vi "Correct_Paths_For_OS_in_XML.vi"(2 "XML Elements":string) -> (0 "String":string)   [LabVIEW 2011]
uses:
  <vilib>/regexp/Match Regular Expression.xnode
panel:
  out "before match":string
  out "Numeric":i32
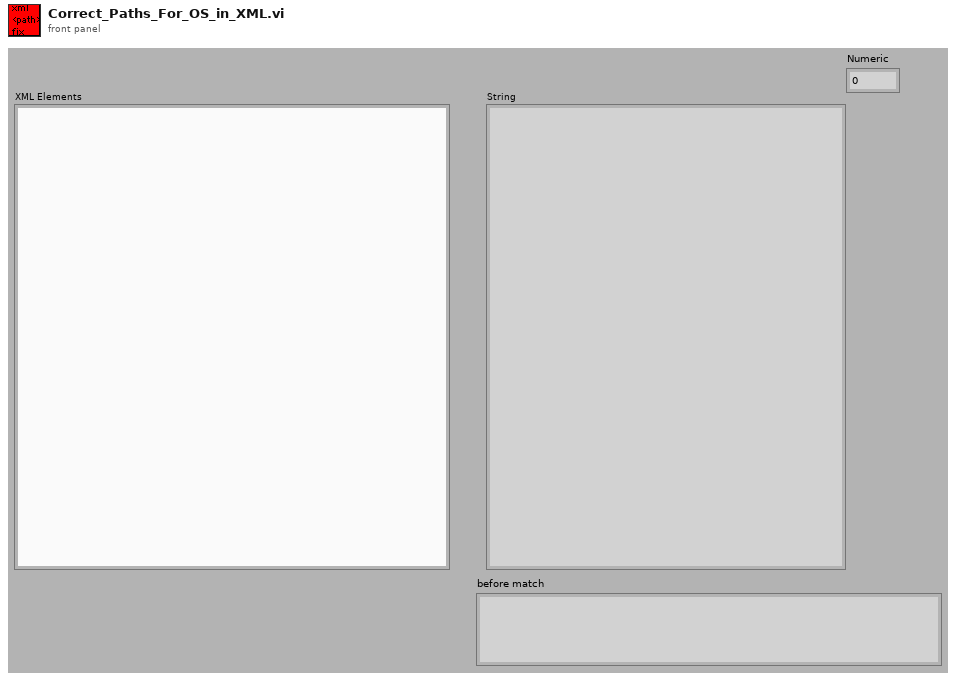
[diagram p1: front panel]
types:
  T1 = enum32{"invalid OS target", "Mac OS", "Windows 3.1", "Windows 95/NT", "Solaris 1", "Solaris 2", "HP-UX", "PowerMAX", "Linux", "Irix", "Rhapsody", "BeOS", "AIX", "OSF1", "VxWorks", "PharLap", "Carbon", "RTX", "Windows x64", "Linux x64"}
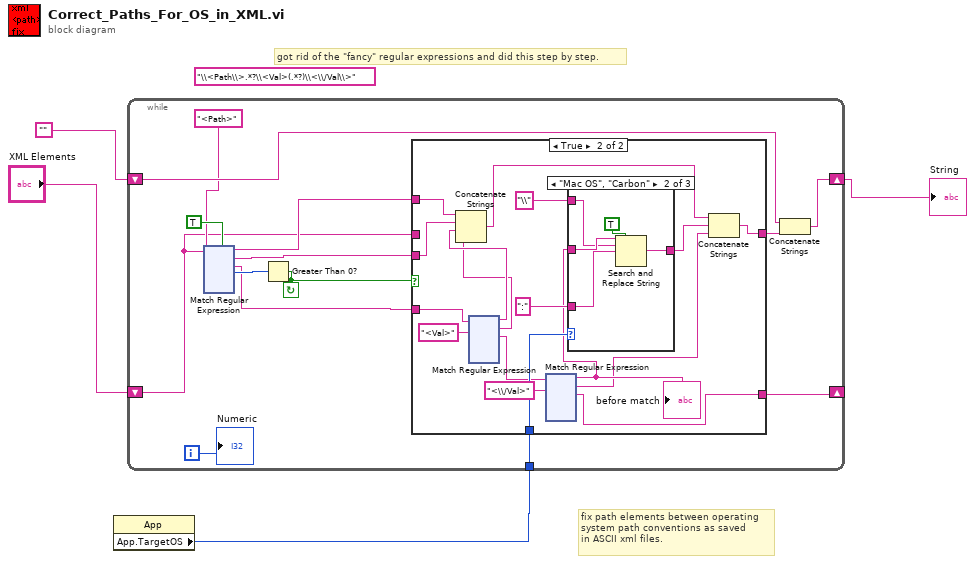
[diagram p0: block diagram]
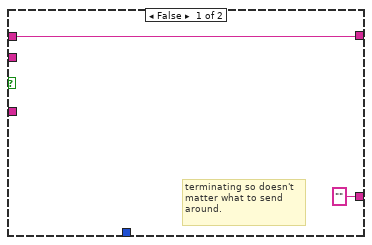
[diagram p2: hidden frame]
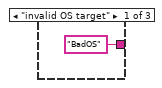
[diagram p3: hidden frame]
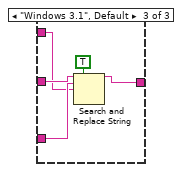
[diagram p4: hidden frame]
diagram:
  (unwired) "\\<Path\\>.*?\\<Val>(.*?)\\<\\/Val\\>"
  # "got rid of the \"fancy\" regular expressions and did this step by step."
  # "fix path elements between operating\nsystem path conventions as saved\nin ASCII xml files."
  n1 = property class="App"() -> ("App.TargetOS"=w2:T1)  [unwired: 2 in, 2 out]
  n2 = while {
    tunnel: w2 -> [w16]
    shift-right: [w5] -> _
    shift-left: "XML Elements" -> [w7]
    shift-right: [w11] -> w4
    shift-left: "" -> [w12]
    i -> [w8]
    stop <- w14 continue-if-true
    n3 = xnode "Match Regular Expression"("input string"=w7, "regular expression"="<Path>", "multiline? (F)"=TRUE) -> ("before match"=w10:string, "whole match"=w17:string, "after match"=w6:string, "offset past match"=w15:i32)  [unwired: 3 in, 2 out]
    n4 = Greater Than 0?(x=w15) -> (x > 0?=w14:bool)
    n5 = case shown="True" w14 {
      tunnel: w17 -> [_ w27]
      tunnel: w16 -> [_ w35]
      tunnel: [w20 w34] -> w13
      tunnel: w7 -> [w20 _]
      tunnel: w10 -> [_ w28]
      tunnel: w6 -> [_ w32]
      tunnel: ["" ("after match") w23] -> w5
      frame False {
        # "terminating so doesn't\nmatter what to send\naround."
      }
      frame True {
        n6 = xnode "Match Regular Expression"("input string"=w32, "regular expression"="<Val>") -> ("before match"=w22:string, "whole match"=w21:string, "after match"=w31:string)  [unwired: 4 in, 3 out]
        n7 = Concatenate Strings(w28, w27, w22, w21) -> (w26:string)
        n8 = xnode "Match Regular Expression"("input string"=w31, "regular expression"="<\\/Val>") -> ("before match"=w29:string, "whole match"=w24:string, "after match"=w23:string)  [unwired: 4 in, 3 out]
        "before match" <- w29
        n9 = case shown="\"Mac OS\", \"Carbon\"" w35 {
          tunnel: w29 -> [_ w269 w272]
          tunnel: "\\" ("search string") -> [_ w268 w270]
          tunnel: ":" ("replace string (\"\")") -> [_ w267 w271]
          tunnel: ["BadOS" ("result string") w266 w273] -> w25
          frame "invalid OS target" {
          }
          frame "Mac OS", "Carbon" {
            n10 = Search and Replace String(replace all?=TRUE ("replace all? (F)"), input string=w269, search string=w268, replace string=w267) -> (result string=w266:string)  [unwired: 4 in, 3 out]
          }
          frame "Windows 3.1", Default {
            n11 = Search and Replace String(replace all?=TRUE ("replace all? (F)"), input string=w272, search string=w271, replace string=w270) -> (result string=w273:string)  [unwired: 4 in, 3 out]
          }
        }
        n12 = Concatenate Strings(w26, w25, w24) -> (w34:string)
      }
    }
    n13 = Concatenate Strings(w12, w13) -> (w11:string)
    "Numeric" <- w8
  }
  "String" <- w4
